vi "13.3 Moments.vi"() -> ()   [LabVIEW 2016]
doc: "This example shows how to use the Edge Tool in NI Vision. The Edge Tool finds edges (or sharp transitions in the pixels values) along a given line or ROI profile. The Edge Tool is a precursor function to many of the gauging and inspection tasks. For example, the location of the edges found along a line profile across an object can interpreted as the boundaries of the object whose dimensions have to be measured for a gauging application or the presence of a crack in the surface of an object for an inspection application."
uses:
  <vilib>/vision/NI_Vision_Development_Module.lvlib
panel:
  out "Img":T1(plugin-control)
  in  "Color":u32[](array[colorbox])=[3381759, 16776770, 16777225, 6618880]
  in  "Overlay Type":u16[](array[ring])=[2, 1, 3, 0] items=["Rectangle", "Numbers", "Points", "Lines"]
  out "Particle Measurements (Pixels)":dbl[][](array[numeric]) format="%.2f"
  in  "Pixel Measurements":T2[](array[typedef])=[0, 1, 2, 3, 42, 8, 9, 10, 11, 4, 5, 6, 7] items=["Center of Mass X", "Center of Mass Y", "First Pixel X", "First Pixel Y", "Bounding Rect Left", "Bounding Rect Top", "Bounding Rect Right", "Bounding Rect Bottom", "Max Feret Diameter Start X", "Max Feret Diameter Start Y", "Max Feret Diameter End X", "Max Feret Diameter End Y", "Max Horiz. Segment Length Left", "Max Horiz. Segment Length Right", "Max Horiz. Segment Length Row", "-", "Bounding Rect Width", "Bounding Rect Height", "Bounding Rect Diagonal", "Perimeter", "Convex Hull Perimeter", "Holes' Perimeter", "Max Feret Diameter", "Equivalent Ellipse Major Axis", "Equivalent Ellipse Minor Axis", "Equivalent Ellipse Minor Axis (Feret)", "Equivalent Rect Long Side", "Equivalent Rect Short Side", "Equivalent Rect Diagonal", "Equivalent Rect Short Side (Feret)", "Average Horiz. Segment Length", "Average Vert. Segment Length", "Hydraulic Radius", "Waddel Disk Diameter", "-", "Area", "Holes' Area", "Particle & Holes' Area", "Convex Hull Area", "Image Area", "-", "Number of Holes", "Number of Horiz. Segments", "Number of Vert. Segments", "-", "Orientation", "Max Feret Diameter Orientation", "-", "% Area/Image Area", "% Area/(Particle & Holes' Area)", "Ratio of Equivalent Ellipse Axes", "Ratio of Equivalent Rect Sides", "-", "Elongation Factor", "Compactness Factor", "Heywood Circularity Factor", "Type Factor", "-", "Sum X", "Sum Y", "Sum XX", "Sum XY", "Sum YY", "Sum XXX", "Sum XXY", "Sum XYY", "Sum YYY", "-", "Moment of Inertia XX", "Moment of Inertia XY", "Moment of Inertia YY", "Moment of Inertia XXX", "Moment of Inertia XXY", "Moment of Inertia XYY", "Moment of Inertia YYY", "Norm. Moment of Inertia XX", "Norm. Moment of Inertia XY", "Norm. Moment of Inertia YY", "Norm. Moment of Inertia XXX", "Norm. Moment of Inertia XXY", "Norm. Moment of Inertia XYY", "Norm. Moment of Inertia YYY", "Hu Moment 1", "Hu Moment 2", "Hu Moment 3", "Hu Moment 4", "Hu Moment 5", "Hu Moment 6", "Hu Moment 7"]
  in  "Threshold":cluster{"Lower\nValue":sgl, "Upper\nValue":sgl}={"Lower\nValue"=0.0, "Upper\nValue"=128.0}
  in  "Stop":bool
  # "Instructions:\n1.Select Pixel Mesurements.\n2.Match the Overlay Type to the selected pixel mesurements.\n3. Match the display color to the overlay type.\n\n\nEvery overlay Type extract data for display from pixel mesurements.\n\nClass of Overlay Type:\n1. Rectangle: (left,top,right, bottom).\n2. Numbers:(x,y,Number).\n3.Points: (x,y).\n4.Lines:(startX,startY,endX,endY)"
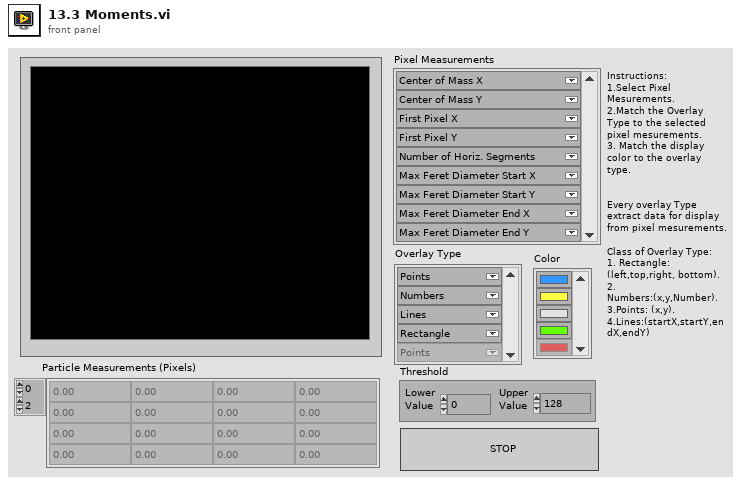
[diagram p1: front panel]
types:
  T1 = typedef "IMAQ Image.ctl" = refnum<image>
  T2 = typedef "Particle Parameters" = i32
  T3 = cluster{"Threshold":cluster{"Lower\nValue":sgl, "Upper\nValue":sgl}, "Pixel Measurements":T2[], "Overlay Type":u16[], "Color":u32[]}
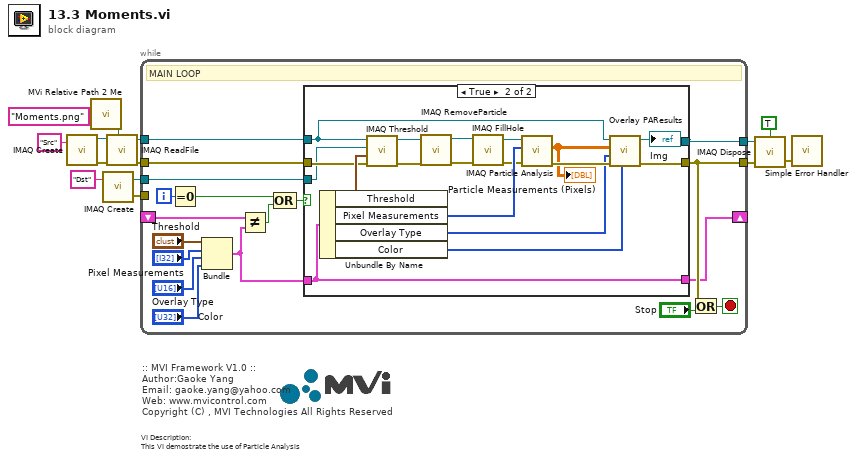
[diagram p0: block diagram]
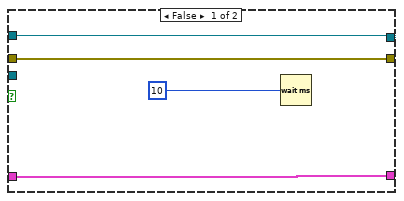
[diagram p2: hidden frame]
diagram:
  # "VI Description:\nThis VI demostrate the use of Particle Analysis"
  # ":: MVI Framework V1.0 ::\nAuthor:Gaoke Yang\nEmail: gaoke.yang@yahoo.com\nWeb: www.mvicontrol.com\nCopyright (C) , MVI Technologies All Rights Reserved"
  n1 = call "IMAQ Create"("Image Name"="Src") -> ("New Image"=w13:T1, "error out"=w12:errorcluster)  [unwired: 4 in]
  n2 = call "MVi Relative Path 2 Me.vi"("Relative Path"="Moments.png" ("name or relative path")) -> ("Appended Dir"=w8:path)  [unwired: 5 in, 1 out]
  n3 = call "IMAQ Create"("Image Name"="Dst") -> ("New Image"=w2:T1, "error out"=w1:errorcluster)  [unwired: 4 in]
  n4 = call "IMAQ ReadFile"("File Path"=w8, "error in (no error)"=w12, "Image"=w13) -> ("error out"=w5:errorcluster, "Image Out"=w4:T1)  [unwired: 4 in, 3 out]
  n5 = while "MAIN LOOP" {
    tunnel: w4 -> [w19]
    tunnel: w5 -> [w18]
    tunnel: [w29] -> w11
    tunnel: [w30] -> w10
    shift-right: [w26] -> _
    shift-left: _ -> [w24]
    tunnel: w2 -> [w20]
    tunnel: w1 -> [_]
    i -> [w28]
    stop <- w31 stop-if-true
    # "MAIN LOOP"
    n6 = Equal To 0?(x=w28) -> (x = 0?=w25:bool)
    n7 = Bundle("Threshold"="Threshold", "Pixel Measurements"="Pixel Measurements", "Overlay Type"="Overlay Type", "Color"="Color") -> (w22:T3)  [unwired: 1 in]
    n8 = Not Equal?(x=w24, y=w22) -> (x != y?=w23:bool)
    n9 = Compound Arithmetic op=OR(w25, w23) -> (w27:bool)
    n10 = case shown="True" w27 {
      tunnel: w18 -> [w35 w52]
      tunnel: w19 -> [w36 w37]
      tunnel: [w36 w46] -> w30
      tunnel: [w35 w47] -> w29
      tunnel: [w34 w54] -> w26
      tunnel: w22 -> [w34 w54]
      tunnel: w20 -> [_ w50]
      frame False {
        n11 = Wait (ms)(milliseconds to wait=u32 10) -> ()  [unwired: 1 out]
      }
      frame True {
        n12 = Unbundle By Name(w54) -> ("Threshold"=w53:cluster{"Lower\nValue":sgl, "Upper\nValue":sgl}, "Pixel Measurements"=w51:T2[], "Overlay Type"=w45:u16[], "Color"=w44:u32[])
        n13 = call "IMAQ Threshold"("error in (no error)"=w52, "Range"=w53, "Image Dst"=w50, "Image Src"=w37) -> ("error out"=w41:errorcluster, "Image Dst Out"=w40:T1)  [unwired: 2 in, 4 out]
        n14 = call "IMAQ RemoveParticle"("error in (no error)"=w41, "Image Src"=w40) -> ("error out"=w42:errorcluster, "Image Dst Out"=w43:T1)  [unwired: 8 in]
        n15 = call "IMAQ FillHole"("error in (no error)"=w42, "Image Src"=w43) -> ("error out"=w39:errorcluster, "Image Dst Out"=w38:T1)  [unwired: 4 in]
        n16 = call "IMAQ Particle Analysis"("error in (no error)"=w39, "Pixel Measurements"=w51, "Image"=w38) -> ("error out"=w49:errorcluster, "Particle Measurements (Pixels)"=w48:dbl[][])  [unwired: 3 in, 4 out]
        "Particle Measurements (Pixels)" <- w48
        n17 = call "Overlay PAResults.vi"("Color"=w44, "error in"=w49, "Overlay Type"=w45, "Particle Measurements (Pixels)"=w48, "Image"=w37) -> ("error out"=w47:errorcluster, "Image Out"=w46:T1)  [unwired: 5 in]
        "Img" <- w46
      }
    }
    n18 = Or(x=w29, y="Stop") -> (x .or. y?=w31:bool)
  }
  n19 = call "IMAQ Dispose"("All Images? (No)"=TRUE, "Image"=w10, "error in (no error)"=w11) -> ("error out"=w7:errorcluster)  [unwired: 3 in]
  n20 = call <vilib>:"Simple Error Handler.vi"("error in (no error)"=w7) -> ()  [unwired: 4 in, 5 out]
